vi "GetCost.vi"(8 "error in (no error)":errorcluster, 11 "reference in":refnum<class "Equipment.lvclass">) -> (0 "error out":errorcluster, 2 "Cost":dbl, 3 "reference out":refnum<class "Equipment.lvclass">)   [LabVIEW 2020, in "Equipment.lvclass"]
uses:
  Equipment.lvclass
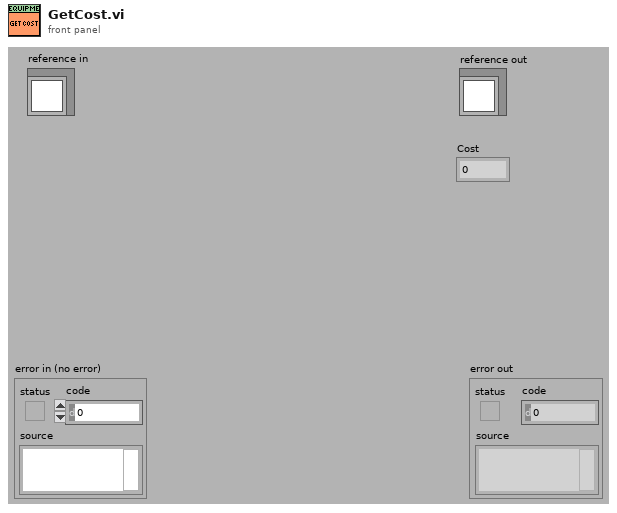
[diagram p1: front panel]
types:
  T1 = typedef "Equipment.lvclass/ObjectAttributes.ctl" = cluster{"ID":string, "Cost":dbl}
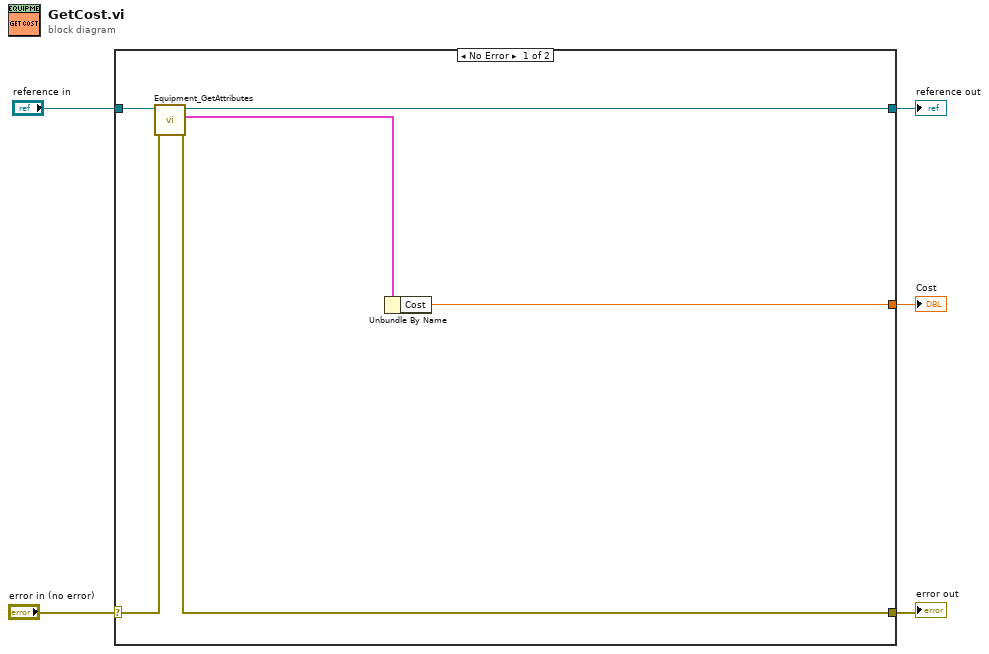
[diagram p0: block diagram]
diagram:
  n1 = case shown="No Error" "error in (no error)" {
    selector: "error in (no error)" -> [w11 w13]
    tunnel: [w9 w13] -> w4
    tunnel: [w7 w12] -> w2
    tunnel: "reference in" -> [w8 w12]
    tunnel: [w6 _] -> w1
    frame No Error {
      n2 = call "Equipment_GetAttributes.vi"("error in (no error)"=w11, "reference in"=w8) -> ("error out"=w9:errorcluster, "Data"=w10:T1, "reference out"=w7:refnum<class "Equipment.lvclass">)  [unwired: 6 in, 1 out]
      n3 = Unbundle By Name(w10) -> ("Cost"=w6:dbl)
    }
    frame Error {
    }
  }
  "error out" <- w4
  "reference out" <- w2
  "Cost" <- w1
